vi "niRFUtil WFM Complex N Differential.vi"(7 "Waveform In":T1 {"y" format="%.2f"; "dx" format="%^.2e"; "x0" format="%^.2e"}, 13 "N":i16=1) -> (8 "Waveform Out":T1 {"y" format="%.2f"; "dx" format="%^.2e"; "x0" format="%^.2e"})   [LabVIEW 2015, in "niRFUtil.lvlib"]
doc: "(c) Copyright 2006, National Instruments, Inc. This VI may not be duplicated, sold, or distributed without written consent from National Instruments."
uses:
  niRFUtil.lvlib
  Includes/niRFUtil INC Complex Waveform.ctl
  Includes/niRFUtil INC Complex Array.ctl
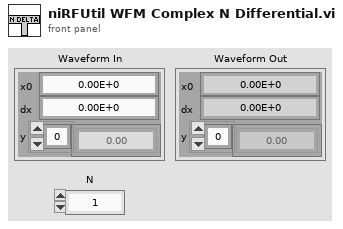
[diagram p1: front panel]
types:
  T1 = typedef "niRFUtil.lvlib/niRFUtil INC Complex Waveform.ctl" = cluster{"x0":dbl, "dx":dbl, "y":T2}
  T2 = typedef "niRFUtil.lvlib/niRFUtil INC Complex Array.ctl" = csg[]
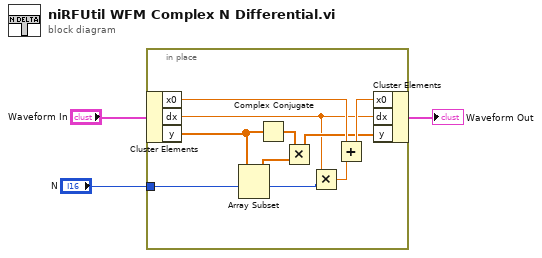
[diagram p0: block diagram]
diagram:
  n1 = in-place {
    in-place-border: "N" -> [w6]
    n2 = in-place-cluster #1("Waveform In") -> ("x0"=w11:dbl, "dx"=w7:dbl, "y"=w10:T2)
    n3 = Array Subset(array=w10, index=w6) -> (w5:T2)  [unwired: 1 in]
    n4 = Complex Conjugate(1:w10) -> (0:w12:T2)
    n5 = Multiply(x=w12, y=w5) -> (x*y=w8:T2)
    n6 = Multiply(x=w7, y=w6) -> (x*y=w4:dbl)
    n7 = Add(x=w11, y=w4) -> (x+y=w9:dbl)
    n8 = in-place-cluster #1("x0"=w9, "dx"=w7, "y"=w8) -> (→"Waveform Out":T1)
  }
